vi "PUT Sum.vi"(0 "Sum":dbl) -> ()   [LabVIEW 2013]
uses:
  Action.ctl
  Sensor State FGV Selector.ctl
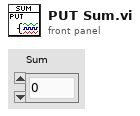
[diagram p1: front panel]
types:
  T1 = typedef "Sensor State FGV Selector.ctl" = enum16{"X Position", "Y Position", "Z Position", "Sum", "Division"}
  T2 = typedef "Action.ctl" = enum16{"GET", "PUT", "DELETE"}
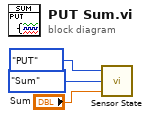
[diagram p0: block diagram]
diagram:
  n1 = call "Sensor State.vi"("Input"="Sum", "Sensor State FGV Selector"=Sensor_State_FGV_Selector."Sum", "Action"=Action."PUT") -> ()  [unwired: 1 out]
